vi "Place Front Gear.vi"(8 "error in":errorcluster) -> (0 "error out":errorcluster)   [LabVIEW 2016]
uses:
  Refname/Motors.ctl
  Refname/Refname to String (Motors).vi
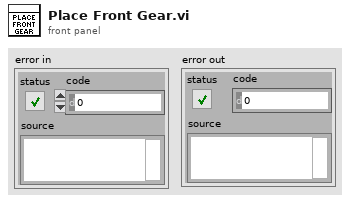
[diagram p1: front panel]
types:
  T1 = typedef "Motors.ctl" = enum16{"Wheel 1", "Swerve 1", "Wheel 2", "Swerve 2", "Wheel 3", "Swerve 3", "Wheel 4", "Swerve 4", "Climber"}
  T2 = typedef "WPI_MotorControlDeviceRef.ctl" = cluster{"DeviceStatus":errorcluster, "Type":T3, "PWM":cluster{"PWM Channel":T4, "DeadBand":T5}, "CAN":cluster{"Device Number":u8, "SetOutput VI Ref":variant, "GetOutput VI Ref":variant, "Enable VI Ref":variant, "Disable VI Ref":variant, "Data":variant}, "Invert":bool}
  T3 = typedef "WPI_MotorControlType.ctl" = enum16{"PWM", "CAN"}
  T4 = typedef "FPGA_DIOPWMChannel.ctl" = enum8{"PWM 0", "PWM 1", "PWM 2", "PWM 3", "PWM 4", "PWM 5", "PWM 6", "PWM 7", "PWM 8", "PWM 9", "PWM MXP 0", "PWM MXP 1", "PWM MXP 2", "PWM MXP 3", "PWM MXP 4", "PWM MXP 5", "PWM MXP 6", "PWM MXP 7", "PWM MXP 8", "PWM MXP 9", "Invalid"}
  T5 = typedef "WPI_PWMDeadband.ctl" = cluster{"Name":string, "maxPositivePwm":i32, "minPositivePwm":i32, "centerPwm":i32, "maxNegativePwm":i32, "minNegativePwm":i32, "angularRange":u16}
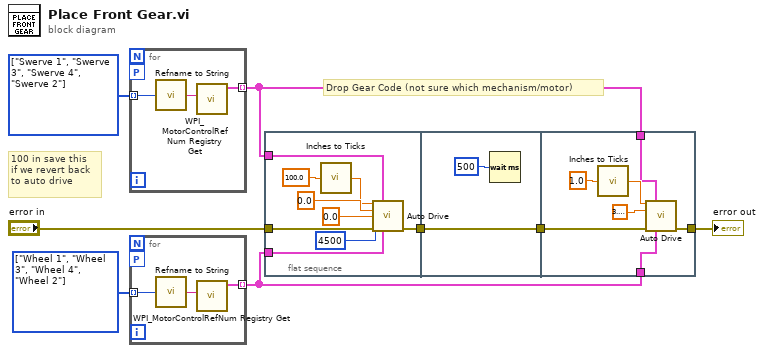
[diagram p0: block diagram]
diagram:
  w7 = T1[] [enum."Wheel 1", enum."Wheel 3", enum."Wheel 4", enum."Wheel 2"] items=["Wheel 1", "Swerve 1", "Wheel 2", "Swerve 2", "Wheel 3", "Swerve 3", "Wheel 4", "Swerve 4", "Climber"]
  w8 = T1[] [enum."Swerve 1", enum."Swerve 3", enum."Swerve 4", enum."Swerve 2"] items=["Wheel 1", "Swerve 1", "Wheel 2", "Swerve 2", "Wheel 3", "Swerve 3", "Wheel 4", "Swerve 4", "Climber"]
  # "100 in save this\nif we revert back \nto auto drive"
  # "Drop Gear Code (not sure which mechanism/motor)"
  n1 = for {
    workers-P: _ -> [_]
    tunnel: w8 -> [w11] mode=indexing
    tunnel: [w9] -> w5 mode=indexing
    n2 = call-poly "Refname to String.vi"("Enum"=w11) -> ("String"=w10:string)
    n3 = call <vilib>:"WPI_MotorControlRefNum Registry Get.vi"("refnum name"=w10) -> ("MotorControlDevRef"=w9:T2)  [unwired: 9 in, 1 out]
  }
  n4 = for {
    workers-P: _ -> [_]
    tunnel: w7 -> [w14] mode=indexing
    tunnel: [w12] -> w4 mode=indexing
    n5 = call-poly "Refname to String.vi"("Enum"=w14) -> ("String"=w13:string)
    n6 = call <vilib>:"WPI_MotorControlRefNum Registry Get.vi"("refnum name"=w13) -> ("MotorControlDevRef"=w12:T2)  [unwired: 9 in, 1 out]
  }
  n7 = flat-sequence {
    tunnel: w5 -> [w23]
    tunnel: w4 -> [w19]
    tunnel: "error in" -> [w21]
    tunnel: [w20] -> w2
    tunnel: w2 -> [w25]
    tunnel: [w25] -> w1
    tunnel: [w30] -> w6
    tunnel: w5 -> [w29]
    tunnel: w4 -> [w28]
    tunnel: w1 -> [w26]
    frame #0 {
      n8 = call "Inches to Ticks.vi"("Inches"=100.0 ("Ticks(Distance)")) -> ("Ticks"=w17:dbl)
      n9 = call "Auto Drive.vi"("Ticks(Distance)"=w17, "Swerve DevRef"=w23, "Drive Angle"=0.0, "Start Power"=0.0, "Time Condition"=u32 4500, "error in"=w21, "Wheel DevRef"=w19) -> ("error out"=w20:errorcluster)  [unwired: 8 in]
    }
    frame #1 {
      n10 = Wait (ms)(milliseconds to wait=u32 500) -> ()  [unwired: 1 out]
    }
    frame #2 {
      n11 = call "Inches to Ticks.vi"("Inches"=1.0) -> ("Ticks"=w31:dbl)
      n12 = call "Auto Drive.vi"("Ticks(Distance)"=w31, "Swerve DevRef"=w29, "Drive Angle"=3.141592653589793, "error in"=w26, "Wheel DevRef"=w28) -> ("error out"=w30:errorcluster)  [unwired: 10 in]
    }
  }
  "error out" <- w6
